vi "Generate Single Overlay Text.vi"(8 "error in":errorcluster, 10 "Overlay":T1, 11 "BigMAQ in":refnum<class "BigMAQ.lvclass">) -> (0 "error out":errorcluster, 3 "BigMAQ out":refnum<class "BigMAQ.lvclass">)   [LabVIEW 2019, in "BigMAQ.lvclass"]
uses:
  BigMAQ.lvclass
  Overlay.ctl
  BigMAQ.lvclass/BigMAQ.ctl
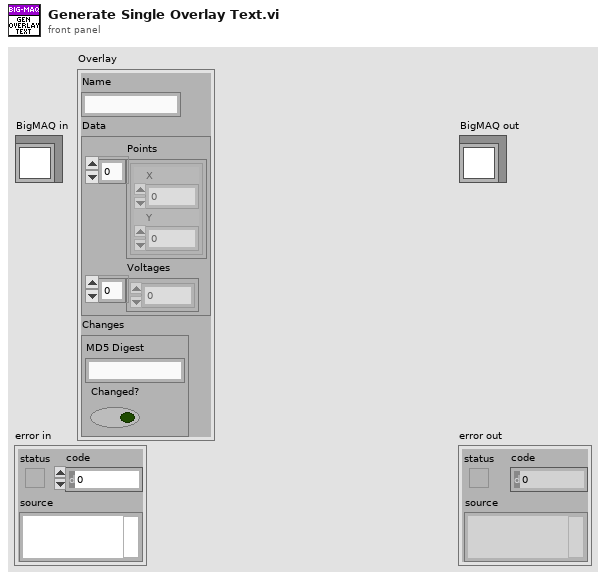
[diagram p1: front panel]
types:
  T1 = typedef "BigMAQ.lvclass/Overlay.ctl" = cluster{"Name":string, "Data":cluster{"Points":cluster{"X":dbl, "Y":dbl}[], "Voltages":dbl[]}, "Changes":cluster{"MD5 Digest":string, "Changed?":bool}}
  T2 = cluster{"Desired Font (Application)":enum16{"User-specified Font", "Application Font", "System Font", "Dialog Font"}, "[User-specified Font]":cluster{"Font Name":string, "Size":i16, "Strikeout?":bool, "Italic?":bool, "Underline?":bool, "Outline?":bool, "Shadow?":bool, "Bold?":bool, "Rotation Angle":dbl}, "Horizontal Alignment":i16, "Vertical Alignment":i16}
  T3 = typedef "IMAQ Image.ctl" = refnum<image>
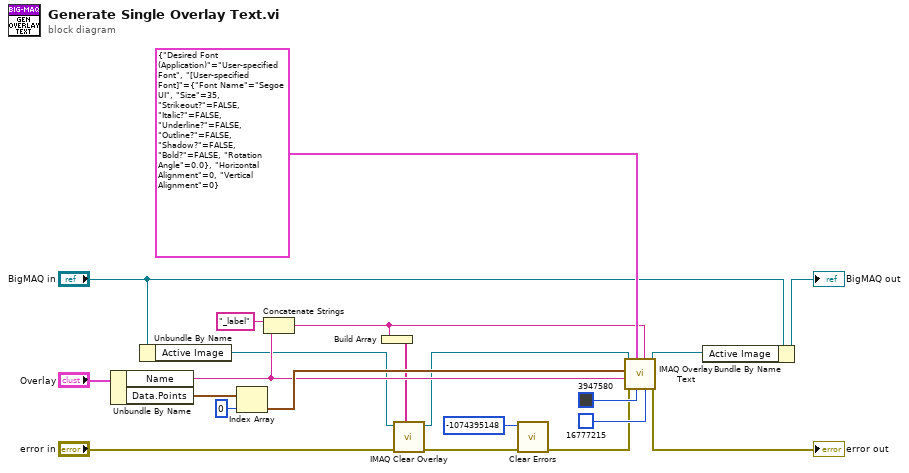
[diagram p0: block diagram]
diagram:
  n1 = Unbundle By Name("Overlay") -> ("Name"=w11:string, "Data.Points"=w19:cluster{"X":dbl, "Y":dbl}[])
  n2 = Unbundle By Name("BigMAQ in") -> ("Active Image"=w9:T3)
  n3 = Index Array(array=w19, index=0) -> (element=w17:cluster{"X":dbl, "Y":dbl})
  n4 = Concatenate Strings("_label" ("string"), w11) -> (w8:string)
  n5 = Build Array(w8) -> (w7:string[])
  n6 = call "IMAQ Clear Overlay"("Groups"=w7, "error in (no error)"="error in", "Image"=w9) -> ("error out"=w5:errorcluster, "Image Out"=w2:T3)  [unwired: 7 in]
  n7 = call <vilib>:"Clear Errors.vi"("error in (no error)"=w5, "specific error code to clear (0: all)"=-1074395148) -> ("error out"=w4:errorcluster)  [unwired: 4 in, 1 out]
  n8 = call "IMAQ Overlay Text"("BG Color (Transparent)"=u32 16777215, "Group"=w8, "Text Color (black)"=u32 3947580, "Font, Size & Style"=T2 {"Desired Font (Application)"=enum."User-specified Font", "[User-specified Font]"={"Font Name"="Segoe UI", "Size"=35, "Strikeout?"=FALSE, "Italic?"=FALSE, "Underline?"=FALSE, "Outline?"=FALSE, "Shadow?"=FALSE, "Bold?"=FALSE, "Rotation Angle"=0.0}, "Horizontal Alignment"=0, "Vertical Alignment"=0}, "error in (no error)"=w4, "String"=w11, "Origin"=w17, "Image"=w2) -> ("error out"=→"error out":errorcluster, "Image Out"=w1:T3)  [unwired: 2 in]
  n9 = Bundle By Name(cluster="BigMAQ in", "Active Image"=w1) -> (→"BigMAQ out":refnum<class "BigMAQ.lvclass">)
